vi "Log INFO.vi"(7 "Logger Name":string, 8 "error in (no error)":errorcluster, 11 "Message":string) -> (0 "error out":errorcluster)   [LabVIEW 2020, in "Global_logger.lvlib"]
uses:
  Global_logger.lvlib
  Levels.ctl
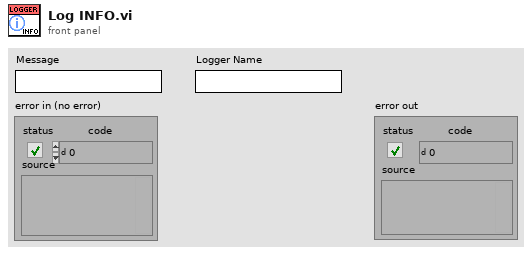
[diagram p1: front panel]
types:
  T1 = typedef "Global_logger.lvlib/Levels.ctl" = enum16{"ALL", "TRACE", "DEBUG", "INFO", "WARN", "ERROR", "FATAL", "OFF"}
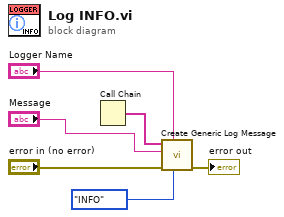
[diagram p0: block diagram]
diagram:
  n1 = Call Chain() -> (call chain=w3:string[])
  n2 = call "Create Generic Log Message.vi"("Level"=Levels."INFO", "Logger Name"="Logger Name", "error in (no error)"="error in (no error)", "Message"="Message", "Call Chain"=w3) -> ("error out"=→"error out":errorcluster)  [unwired: 6 in]
